vi "Do Something.vi"(8 "error in (no error)":errorcluster, 10 "Bytes to Read":i32, 11 "Inst.SPC in":refnum<class "Inst.SPC.lvclass">) -> (0 "error out":errorcluster, 3 "Inst.SPC out":refnum<class "Inst.SPC.lvclass">)   [LabVIEW 2019, in "Inst.SPC.lvclass"]
uses:
  Inst.SPC.lvclass
  67792bfe-8e2c-4879-abc2-cb448bcec168.vi
  Typedefs/Inst.SPC.Commands--Enum.ctl
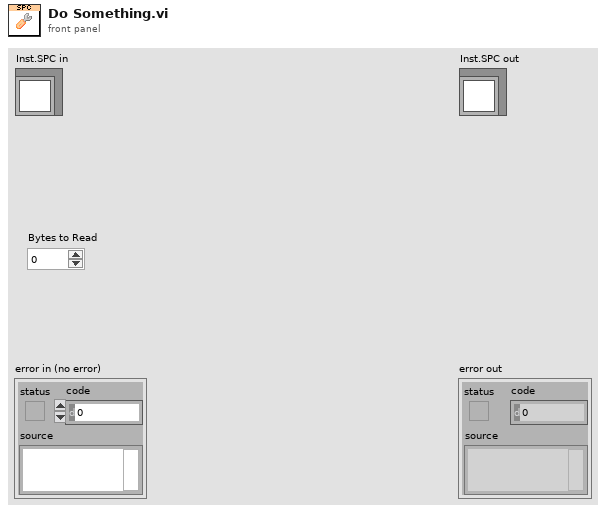
[diagram p1: front panel]
types:
  T1 = typedef "Inst.SPC.lvclass/Inst.SPC.Commands--Enum.ctl" = enum16{"Do Something"}
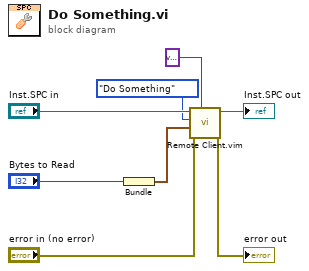
[diagram p0: block diagram]
diagram:
  n1 = Bundle("Bytes to Read"="Bytes to Read") -> (w2:cluster{"Bytes to Read":i32})  [unwired: 1 in]
  n2 = call "Remote Client.vim"("Data Out type"=variant, "error in (no error)"="error in (no error)", "params"=w2, "method"=Inst.SPC.Commands--Enum."Do Something" ("Commands"), "Instrument in"="Inst.SPC in") -> ("error out"=→"error out":errorcluster, "Instrument out"=→"Inst.SPC out":refnum<class "Inst.SPC.lvclass">)  [unwired: 3 in, 2 out]
